vi "robot scara.vi"() -> ()   [LabVIEW 2013]
uses:
  <vilib>/Native 3D Graph/xcontrol/3DPC_SurfacePlot.xctl
panel:
  in  "Sz":dbl(slide) scale=0.0..10.0
  in  "s3":dbl(slide) max=1.4285714285714286 scale=0.0..2.0408163265306123
  in  "xy":dbl(knob) scale=0.0..360.0
  in  "xy2":dbl(knob) scale=-175.0..175.0
  out "3D Graph":refnum<class "Base Datatype.lvclass">[](xcontrol)
  in  "s1":dbl
  in  "s2":dbl
  in  "stop":bool
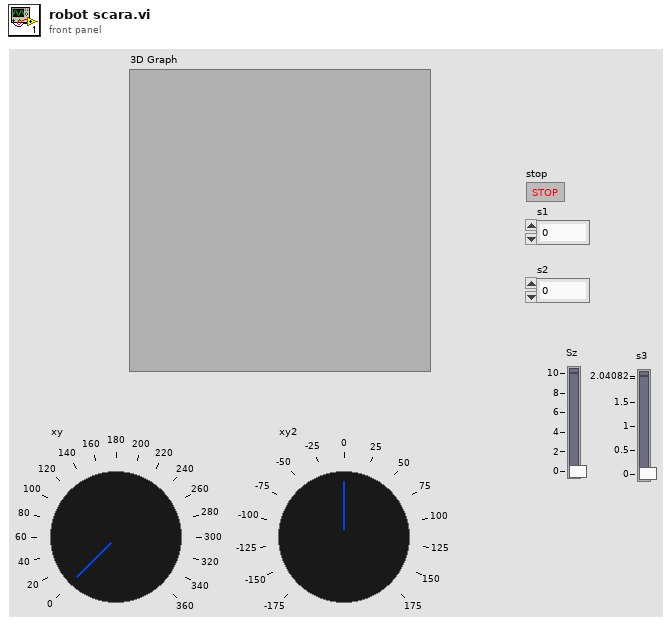
[diagram p1: front panel]
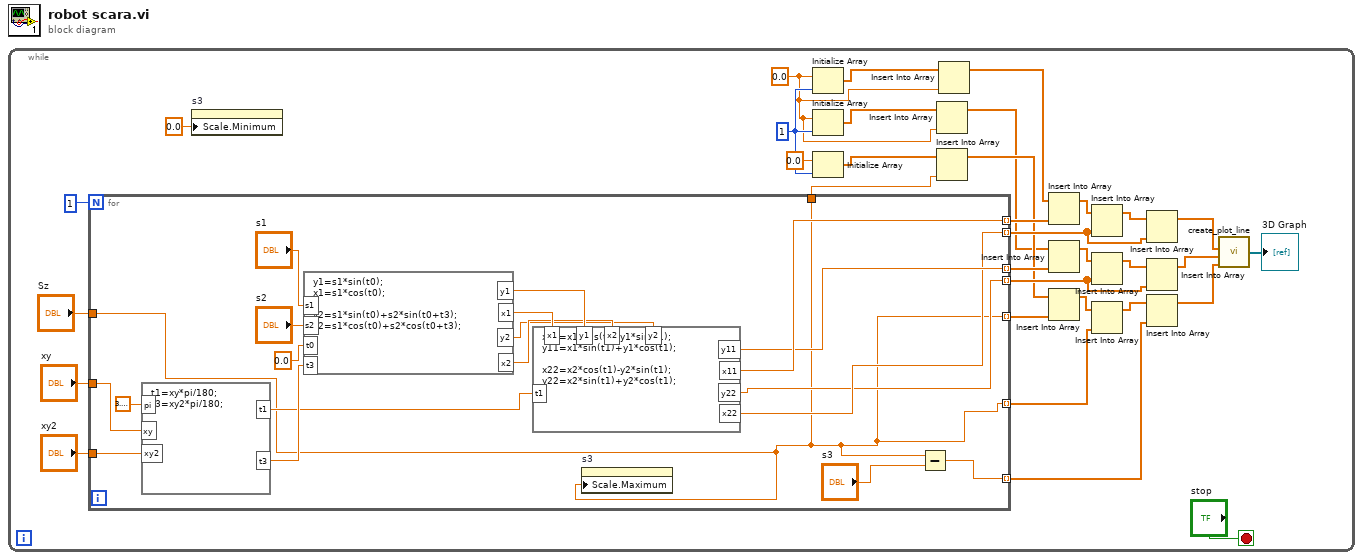
[diagram p0: block diagram]
diagram:
  n1 = while {
    stop <- "stop" stop-if-true
    w1 = 0.0
    w10 = 1 ("dimension size")
    n2 = for {
      N: 1 -> [_]
      tunnel: "xy" -> [w51]
      tunnel: "xy2" -> [w50]
      tunnel: [w38] -> w16 mode=indexing
      tunnel: [w40] -> w25 mode=indexing
      tunnel: [w37] -> w17 mode=indexing
      tunnel: [w39] -> w24 mode=indexing
      tunnel: [w34] -> w23 mode=indexing
      tunnel: [w34] -> w22 mode=indexing
      tunnel: [w35] -> w18 mode=indexing
      tunnel: "Sz" -> [w34]
      tunnel: [w34] -> w8
      n3 = formula code="t1=xy*pi/180;\nt3=xy2*pi/180;"("pi"=3.141592653589793, "xy"=w51, "xy2"=w50) -> ("t1"=w43:dbl, "t3"=w48:dbl)
      n4 = formula code="y1=s1*sin(t0);\nx1=s1*cos(t0);\n\ny2=s1*sin(t0)+s2*sin(t0+t3);\nx2=s1*cos(t0)+s2*cos(t0+t3);"("t0"=0.0 ("input variable"), "s1"="s1", "s2"="s2", "t3"=w48) -> ("y1"=w44:dbl, "x1"=w45:dbl, "y2"=w41:dbl, "x2"=w42:dbl)
      n5 = formula code="x11=x1*cos(t1)-y1*sin(t1);\ny11=x1*sin(t1)+y1*cos(t1);\n\nx22=x2*cos(t1)-y2*sin(t1);\ny22=x2*sin(t1)+y2*cos(t1);"("x1"=w45, "y1"=w44, "t1"=w43, "x2"=w42, "y2"=w41) -> ("y11"=w39:dbl, "x11"=w40:dbl, "y22"=w37:dbl, "x22"=w38:dbl)
      n6 = property on="s3" class="Slide (strict)"("Scale.Maximum"=w34) -> ()  [unwired: 2 in, 2 out]
      n7 = Subtract(x=w34, y="s3") -> (x-y=w35:dbl)
    }
    n8 = property on="s3" class="Slide (strict)"("Scale.Minimum"=0.0 ("Scale.Range:Minimum")) -> ()  [unwired: 2 in, 2 out]
    n9 = Initialize Array(w1, w10) -> (w5:dbl[])
    n10 = Initialize Array(w1, w10) -> (w6:dbl[])
    n11 = Initialize Array(0.0 ("element"), w10) -> (w7:dbl[])
    n12 = Insert Into Array(array=w6, new element=w1) -> (w2:dbl[])  [unwired: 1 in]
    n13 = Insert Into Array(array=w7, new element=w8) -> (w4:dbl[])  [unwired: 1 in]
    n14 = Insert Into Array(array=w5, new element=w1) -> (w3:dbl[])  [unwired: 1 in]
    n15 = Insert Into Array(array=w3, new element=w25) -> (w26:dbl[])  [unwired: 1 in]
    n16 = Insert Into Array(array=w2, new element=w24) -> (w27:dbl[])  [unwired: 1 in]
    n17 = Insert Into Array(array=w4, new element=w23) -> (w28:dbl[])  [unwired: 1 in]
    n18 = Insert Into Array(array=w26, new element=w16) -> (w21:dbl[])  [unwired: 1 in]
    n19 = Insert Into Array(array=w27, new element=w17) -> (w20:dbl[])  [unwired: 1 in]
    n20 = Insert Into Array(array=w28, new element=w22) -> (w19:dbl[])  [unwired: 1 in]
    n21 = Insert Into Array(array=w21, new element=w16) -> (w15:dbl[])  [unwired: 1 in]
    n22 = Insert Into Array(array=w20, new element=w17) -> (w14:dbl[])  [unwired: 1 in]
    n23 = Insert Into Array(array=w19, new element=w18) -> (w13:dbl[])  [unwired: 1 in]
    n24 = call <vilib>:"create_plot_line.vi"("z vector"=w13, "y vector"=w14, "x vector"=w15) -> ("plots out"=→"3D Graph":refnum<class "Base Datatype.lvclass">[])  [unwired: 2 in, 6 out]
  }
